vi "VI Tree.vi"   [LabVIEW 2022 SP3, in "VI-Snippet.lvlib"]
uses:
  VI-Snippet.lvlib
  Snippet.ctl
types:
  T1 = typedef "VI-Snippet.lvlib/Snippet.ctl" = cluster{"Image":cluster{"image type":i32, "image depth":i32, "image":u8[], "mask":u8[], "colors":u32[], "Rectangle":cluster{"left":i16, "top":i16, "right":i16, "bottom":i16}}, "niVI":string}
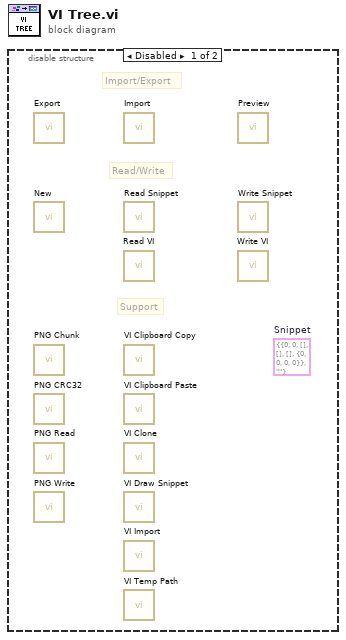
[diagram p0: block diagram]
diagram:
  n1 = disable-structure shown="Disabled" {
    frame Disabled {
      (unwired) T1 {"Image"={"image type"=0, "image depth"=0, "image"=[], "mask"=[], "colors"=[], "Rectangle"={"left"=0, "top"=0, "right"=0, "bottom"=0}}, "niVI"=""}  # Snippet
      # "Import/Export"
      # "Read/Write"
      # "Support"
      n2 = call "Export.vi"() -> ()  [unwired: 10 in, 2 out]
      n3 = call "New.vi"() -> ()  [unwired: 10 in, 2 out]
      n4 = call "PNG Chunk.vi"() -> ()  [unwired: 11 in, 1 out]
      n5 = call "PNG CRC32.vi"() -> ()  [unwired: 11 in, 1 out]
      n6 = call "PNG Read.vi"() -> ()  [unwired: 9 in, 3 out]
      n7 = call "PNG Write.vi"() -> ()  [unwired: 10 in, 2 out]
      n8 = call "Import.vi"() -> ()  [unwired: 9 in, 3 out]
      n9 = call "Read Snippet.vi"() -> ()  [unwired: 10 in, 2 out]
      n10 = call "Read VI.vi"() -> ()  [unwired: 10 in, 2 out]
      n11 = call "VI Clipboard Copy.vi"() -> ()  [unwired: 10 in, 2 out]
      n12 = call "VI Clipboard Paste.vi"() -> ()  [unwired: 10 in, 2 out]
      n13 = call "VI Clone.vi"() -> ()  [unwired: 10 in, 2 out]
      n14 = call "VI Draw Snippet.vi"() -> ()  [unwired: 9 in, 3 out]
      n15 = call "VI Import.vi"() -> ()  [unwired: 9 in, 3 out]
      n16 = call "VI Temp Path.vi"() -> ()  [unwired: 11 in, 1 out]
      n17 = call "Preview.vi"() -> ()  [unwired: 8 in, 4 out]
      n18 = call "Write Snippet.vi"() -> ()  [unwired: 11 in, 1 out]
      n19 = call "Write VI.vi"() -> ()  [unwired: 11 in, 1 out]
    }
    frame Enabled {
    }
  }
